vi "Rect Window Frequency Response.vi"(8 "N":i32, 11 "f":dbl) -> (3 "H(f)":cdb format="%.2f")   [LabVIEW 2021]
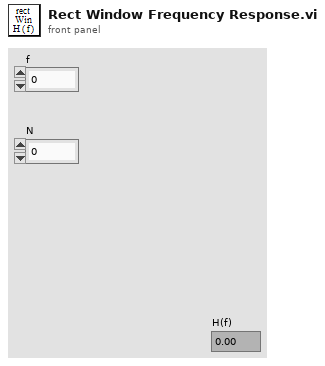
[diagram p1: front panel]
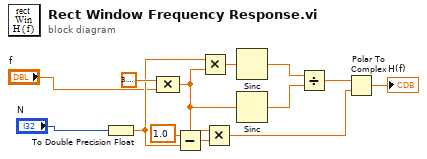
[diagram p0: block diagram]
diagram:
  n1 = To Double Precision Float(number="N") -> (double precision float=w3:dbl)
  n2 = Compound Arithmetic op=MULTIPLY(3.141592653589793 ("Pi"), "f") -> (w6:dbl)
  n3 = Subtract(x=1.0, y=w3) -> (x-y=w4:dbl)
  n4 = Multiply(x=w3, y=w6) -> (x*y=w9:dbl)
  n5 = Multiply(x=w6, y=w4) -> (x*y=w11:dbl)
  n6 = Sinc(1:w9) -> (0:w8:dbl)
  n7 = Sinc(1:w6) -> (0:w7:dbl)
  n8 = Divide(x=w8, y=w7) -> (x/y=w13:dbl)
  n9 = Polar To Complex(1:w11, 2:w13) -> (0:→"H(f)":cdb)
